vi "HeaterControl.vi"() -> ()   [LabVIEW 2025]
doc: "Author: Scott Hannahs <sth@magnet.fsu.edu>\n\nThis software is licensed for use under the “MIT License\"\nCopyright (c) 2025 Scott Hannahs, sth@sth@magnet.sthnet.net\n\nPermission is hereby granted, free of charge, to any person obtaining a copy of this software and associated documentation files (the \"Software\"), to deal in the Software without restriction, including without limitation the rights to use, copy, modify, merge, publish, distribute, sublicense, and/or sell copies of the Software, and to permit persons to whom the Software is furnished to do so, subject to the following conditions: The above copyright notice and this permission notice shall be included in all copies or substantial portions of the Software.\n\nTHE SOFTWARE IS PROVIDED \"AS IS\", WITHOUT WARRANTY OF ANY KIND, EXPRESS OR IMPLIED, INCLUDING BUT NOT LIMITED TO THE WARRANTIES OF MERCHANTABILITY, FITNESS FOR A PARTICULAR PURPOSE AND NONINFRINGEMENT. IN NO EVENT SHALL THE AUTHORS OR COPYRIGHT HOLDERS BE LIABLE FOR ANY CLAIM, DAMAGES OR OTHER LIABILITY, WHETHER IN AN ACTION OF CONTRACT, TORT OR OTHERWISE, ARISING FROM, OUT OF OR IN CONNECTION WITH THE SOFTWARE OR THE USE OR OTHER DEALINGS IN THE SOFTWARE."
uses:
  GL_MHeaterDisplay.vi
  GL_heaterdisplay.vi
  GL_HeaterOn.vi
  GL_TempDspl.vi
  GL_TempUnits.vi
panel:
  out "unit":enum16{"K", "Ohms", "C", "F"}(ring)
  out "Temperature":dbl=1.0 min=0.0 max=600.0 step=0.01 format="%.3f"
  in  "OK":bool
  out "MANUAL HEATER DISPLAY":dbl(slide) caption="AMP" min=0.0 max=99.0 scale=0.0..5.0
  in  "Heater Input":bool[](array[boolean])
  out "HEATER ON":bool
  out "Heater DIsplay":bool[](array[boolean])
  out "HEATER RANGE":dbl format="%.2f"
  out "Change state bit":bool
  in  "MANUAL HEATER":dbl(slide) caption="AMP" min=0.0 max=990.0 scale=0.0..5.0
  out "MANUAL HEATER SETTING":dbl format="%.2f"
  in  "Manual Heater on 2":bool
  out "Manual Heater on":bool
  # "0/1 -4  -3   -2   -1   M"
  # "MANUAL HEATER"
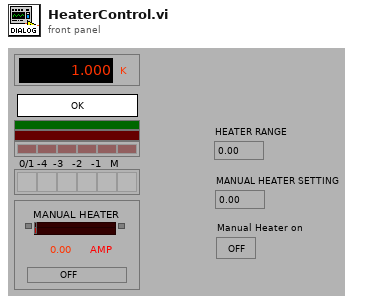
[diagram p1: front panel]
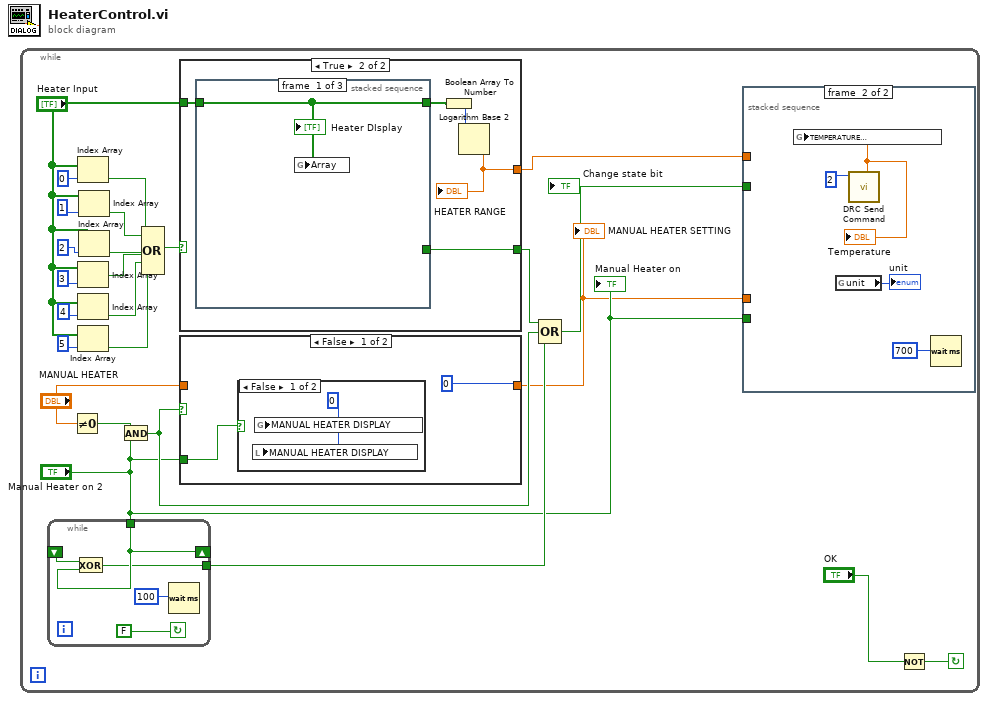
[diagram p0: block diagram]
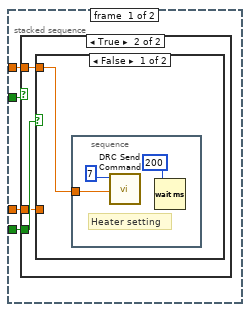
[diagram p2: hidden frame]
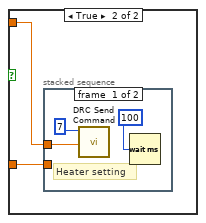
[diagram p4: hidden frame]
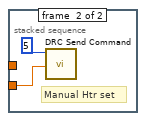
[diagram p5: hidden frame]
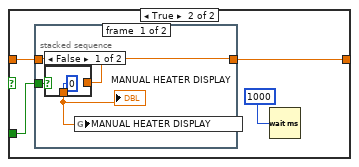
[diagram p7: hidden frame]
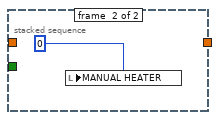
[diagram p9: hidden frame]
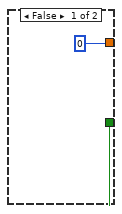
[diagram p10: hidden frame]
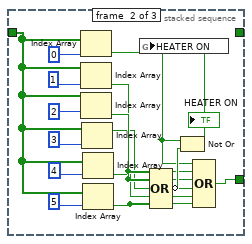
[diagram p11: hidden frame]
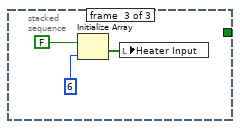
[diagram p12: hidden frame]
diagram:
  n1 = while {
    stop <- w2 continue-if-true
    n2 = while {
      tunnel: [w27] -> w10
      tunnel: "Manual Heater on 2" -> [w28]
      shift-left: _ -> [w30]
      shift-right: [w28] -> _
      stop <- FALSE continue-if-true
      n3 = Exclusive Or(1:w28, 2:w30) -> (0:w27:bool)
      n4 = Wait (ms)(milliseconds to wait=100) -> ()  [unwired: 1 out]
    }
    n5 = Not Equal To 0?(x="MANUAL HEATER") -> (x != 0?=w12:bool)
    n6 = Index Array(array="Heater Input", index=0) -> (element=w19:bool)
    n7 = Index Array(array="Heater Input", index=3) -> (element=w16:bool)
    n8 = Index Array(array="Heater Input", index=4) -> (element=w3:bool)
    n9 = Index Array(array="Heater Input", index=5) -> (element=w4:bool)
    n10 = Index Array(array="Heater Input", index=1) -> (element=w18:bool)
    n11 = Index Array(array="Heater Input", index=2) -> (element=w17:bool)
    n12 = And(x=w12, y="Manual Heater on 2") -> (x .and. y?=w11:bool)
    n13 = Compound Arithmetic op=OR(w19, w18, w17, w16, w3, w4) -> (w20:bool)
    n14 = case shown="True" w20 {
      tunnel: "Heater Input" -> [_ w72]
      tunnel: [FALSE w69] -> w13
      tunnel: [0 w68] -> w8
      frame False {
      }
      frame True {
        n15 = stacked-sequence {
          tunnel: w72 -> [w73 w77 _]
          tunnel: [_ w82 _] -> w69
          tunnel: [w73 _ _] -> w71
          frame #0 {
            n16 = global write "GL_heaterdisplay.vi" "Array"(w73) -> ()
            "Heater DIsplay" <- w73
          }
          frame #1 {
            n17 = Index Array(array=w77, index=0) -> (element=w79:bool)
            n18 = Index Array(array=w77, index=1) -> (element=w80:bool)
            n19 = Index Array(array=w77, index=2) -> (element=w81:bool)
            n20 = Index Array(array=w77, index=3) -> (element=w76:bool)
            n21 = Index Array(array=w77, index=4) -> (element=w74:bool)
            n22 = Index Array(array=w77, index=5) -> (element=w75:bool)
            n23 = Compound Arithmetic op=OR(w80, w81, w76, w74, w75) -> (invert w85:bool)
            n24 = Not Or(1:w85, 2:w79) -> (0:w84:bool)
            "HEATER ON" <- w84
            n25 = global write "GL_HeaterOn.vi" "HEATER ON"(w84) -> ()
            n26 = Compound Arithmetic op=OR(w79, w80, w81, w76, w74, w75) -> (w82:bool)
          }
          frame #2 {
            n27 = Initialize Array(FALSE, 6) -> (w91:bool[])
            n28 = local write "Heater Input"(w91) -> ()
          }
        }
        n29 = Boolean Array To Number(Boolean array=w71) -> (number=w70:u32)
        n30 = Logarithm Base 2(1:w70) -> (0:w68:dbl)
        "HEATER RANGE" <- w68
      }
    }
    n31 = case shown="False" w11 {
      tunnel: "MANUAL HEATER" -> [_ w59]
      tunnel: [0 w58] -> w7
      tunnel: "Manual Heater on 2" -> [w53 w56]
      frame False {
        n32 = case shown="False" w53 {
          frame False {
            w55 = 0
            n33 = local write "MANUAL HEATER DISPLAY"(w55) -> ()
            n34 = global write "GL_MHeaterDisplay.vi" "MANUAL HEATER DISPLAY"(w55) -> ()
          }
          frame True {
          }
        }
      }
      frame True {
        n35 = stacked-sequence {
          tunnel: w59 -> [w62 _]
          tunnel: [w62 _] -> w58
          tunnel: w56 -> [w61 _]
          frame #0 {
            n36 = case shown="False" w61 {
              tunnel: [0 w64] -> w60
              tunnel: w62 -> [_ w64]
              frame False {
              }
              frame True {
              }
            }
            "MANUAL HEATER DISPLAY" <- w60
            n37 = global write "GL_MHeaterDisplay.vi" "MANUAL HEATER DISPLAY"(w60) -> ()
          }
          frame #1 {
            n38 = local write "MANUAL HEATER"(0) -> ()
          }
        }
        n39 = Wait (ms)(milliseconds to wait=1000) -> ()  [unwired: 1 out]
      }
    }
    "MANUAL HEATER SETTING" <- w7
    n40 = Compound Arithmetic op=OR(w13, w11, w10) -> (w14:bool)
    "Change state bit" <- w14
    n41 = stacked-sequence {
      tunnel: w14 -> [w34 _]
      tunnel: "Manual Heater on 2" -> [w33 _]
      tunnel: w8 -> [w32 _]
      tunnel: w7 -> [w31 _]
      frame #0 {
        n42 = case shown="True" w34 {
          tunnel: w33 -> [_ w36]
          tunnel: w32 -> [_ w37]
          tunnel: w31 -> [_ w35]
          frame False {
          }
          frame True {
            n43 = case shown="False" w36 {
              tunnel: w37 -> [w38 w43]
              tunnel: w35 -> [_ w42]
              frame False {
                n44 = stacked-sequence {
                  tunnel: w38 -> [w40]
                  frame #0 {
                    # "Heater setting"
                    n45 = call "DRC Send Command.vi"("Input"=w40, "Command"=7) -> ()  [unwired: 2 in, 3 out]
                    n46 = Wait (ms)(milliseconds to wait=200) -> ()  [unwired: 1 out]
                  }
                }
              }
              frame True {
                n47 = stacked-sequence {
                  tunnel: w43 -> [w45 _]
                  tunnel: w42 -> [_ w47]
                  frame #0 {
                    # "Heater setting"
                    n48 = call "DRC Send Command.vi"("Input"=w45, "Command"=7) -> ()  [unwired: 2 in, 3 out]
                    n49 = Wait (ms)(milliseconds to wait=100) -> ()  [unwired: 1 out]
                  }
                  frame #1 {
                    # "Manual Htr set"
                    n50 = call "DRC Send Command.vi"("Input"=w47, "Command"=5) -> ()  [unwired: 2 in, 3 out]
                  }
                }
              }
            }
          }
        }
      }
      frame #1 {
        n51 = global read "GL_TempUnits.vi" "unit"() -> (→"unit":enum16{"K", "Ohms", "C", "F"})
        n52 = call "DRC Send Command.vi"("Command"=2) -> ("Output"=w50:dbl)  [unwired: 3 in, 2 out]
        "Temperature" <- w50
        n53 = global write "GL_TempDspl.vi" "TEMPERATURE\nDisplay"(w50) -> ()
        n54 = Wait (ms)(milliseconds to wait=700) -> ()  [unwired: 1 out]
      }
    }
    n55 = Not(x="OK") -> (.not. x?=w2:bool)
    "Manual Heater on" <- "Manual Heater on 2"
  }
